vi "MovePossible_MoveComplete.vi"(1 "Axis Array":string[](array[string]), 2 "Position Array":dbl[](array[numeric]), 3 "error in (no error)":errorcluster) -> (8 "Axis moving?":bool[](array[boolean]), 10 "error out":errorcluster)   [LabVIEW 2020]
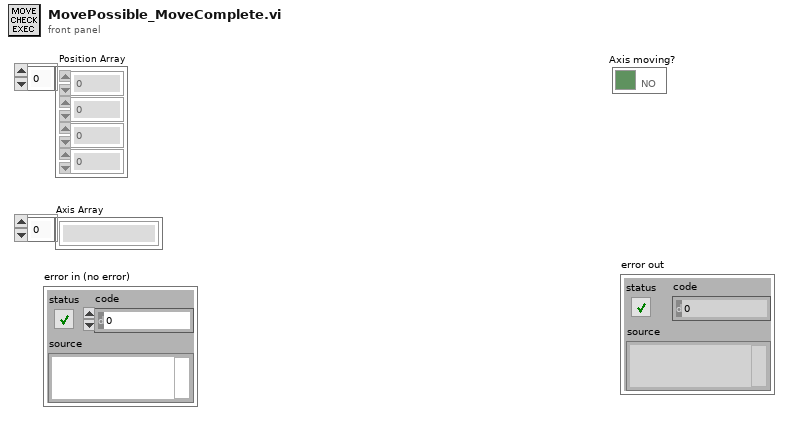
[diagram p1: front panel]
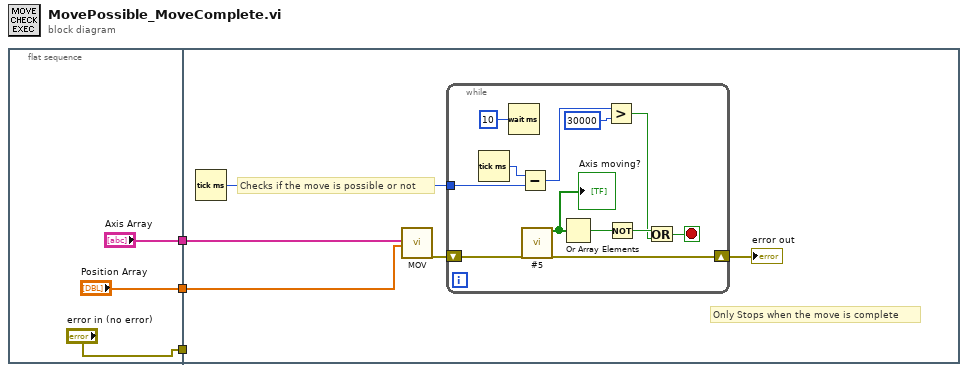
[diagram p0: block diagram]
diagram:
  n1 = flat-sequence {
    tunnel: ["error in (no error)"] -> w3
    tunnel: ["Position Array"] -> w2
    tunnel: ["Axis Array"] -> w1
    tunnel: w3 -> [_]
    tunnel: w2 -> [w9]
    tunnel: w1 -> [w10]
    frame #0 {
    }
    frame #1 {
      # "Checks if the move is possible or not"
      # "Only Stops when the move is complete"
      n2 = Tick Count (ms)() -> (millisecond timer value=w7:u32)
      n3 = call "MOV.vi"("Axes to move"=w10, "Position values"=w9) -> ("error out"=w8:errorcluster)  [unwired: 17 in]
      n4 = while {
        shift-right: [w22] -> w11
        shift-left: w8 -> [w23]
        tunnel: w7 -> [w15]
        stop <- w17 stop-if-true
        n5 = Tick Count (ms)() -> (millisecond timer value=w16:u32)
        n6 = Wait (ms)(milliseconds to wait=u32 10) -> ()  [unwired: 1 out]
        n7 = Subtract(x=w16, y=w15) -> (x-y=w14:u32)
        n8 = call "#5.vi"("error in"=w23) -> ("Axis moving?"=w20:bool[], "error out"=w22:errorcluster)  [unwired: 17 in]
        "Axis moving?" <- w20
        n9 = Or Array Elements(Boolean array=w20) -> (logical OR=w19:bool)
        n10 = Greater?(x=w14, y=u32 30000) -> (0:w13:bool)
        n11 = Not(x=w19) -> (.not. x?=w18:bool)
        n12 = Or(x=w18, y=w13) -> (x .or. y?=w17:bool)
      }
      "error out" <- w11
    }
  }
